vi "Load Project.vi"(8 "error in (no error)":errorcluster, 11 "Application in":refnum<data-value>) -> (0 "error out":errorcluster, 1 "Succeed":bool, 3 "Application out":refnum<data-value>)   [LabVIEW 2015, in "Application.lvclass"]
uses:
  Application.lvclass
  Plugin.lvclass
  Project.lvclass
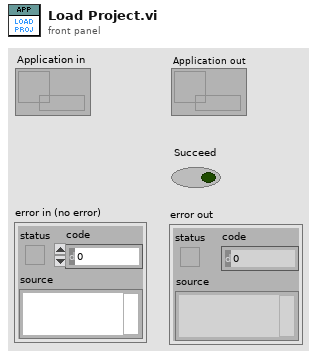
[diagram p1: front panel]
types:
  T1 = typedef "Application Config Typedef.ctl" = cluster{"Auto Load Project":bool, "Project Path":string, "Plugin Folders":string}
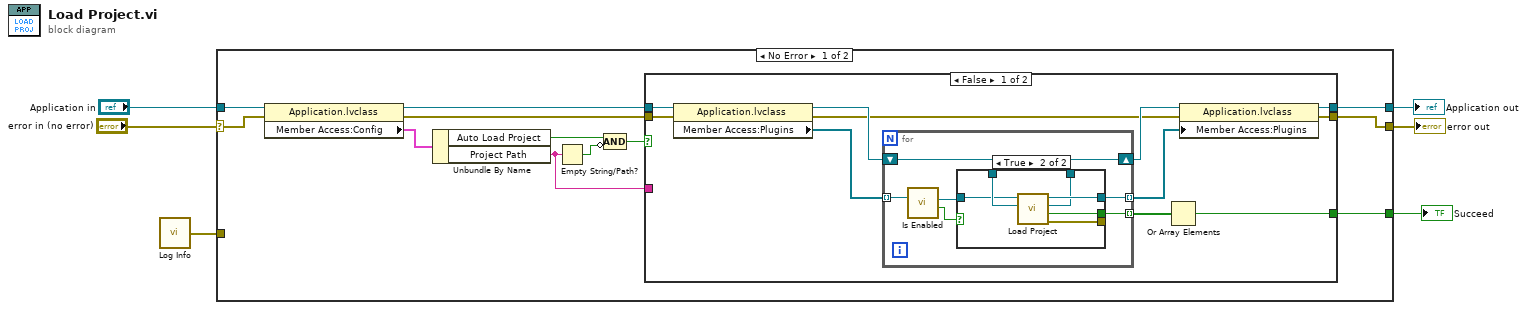
[diagram p0: block diagram]
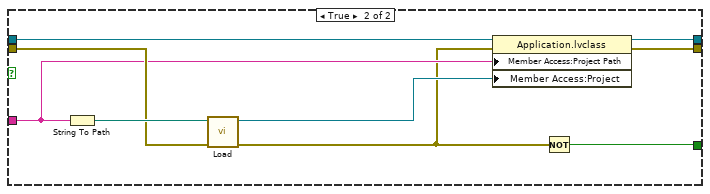
[diagram p3: hidden frame]
diagram:
  n1 = call "Log Info.vi"() -> ("error out"=w4:errorcluster)  [unwired: 5 in]
  n2 = case shown="No Error" "error in (no error)" {
    selector: "error in (no error)" -> [w17 w55]
    tunnel: [w13 w55] -> w5
    tunnel: [w14 w54] -> w2
    tunnel: "Application in" -> [w18 w54]
    tunnel: w4 -> [_ _]
    tunnel: [w12 _] -> w1
    frame No Error {
      n3 = property class="Application.lvclass"(reference=w18, error in=w17) -> (reference out=w16:refnum<data-value>, error out=w15:errorcluster, "Member Access:Config"=w8:T1)
      n4 = Unbundle By Name(w8) -> ("Auto Load Project"=w11:bool, "Project Path"=w7:string)
      n5 = Empty String/Path?(string/path=w7) -> (empty?=w10:bool)
      n6 = Compound Arithmetic op=AND(w11, invert w10) -> (w9:bool)
      n7 = case shown="False" w9 {
        tunnel: w16 -> [w23 w49]
        tunnel: w15 -> [w22 w52]
        tunnel: [w28 w46] -> w14
        tunnel: [w26 w45] -> w13
        tunnel: [w24 w47] -> w12
        tunnel: w7 -> [_ w51]
        frame False {
          n8 = property class="Application.lvclass"(reference=w23, error in=w22) -> (reference out=w20:refnum<data-value>, error out=w19:errorcluster, "Member Access:Plugins"=w21:refnum<class "Plugin.lvclass">[])
          n9 = for {
            tunnel: w21 -> [w32] mode=indexing
            shift-right: [w34] -> w29
            shift-left: w20 -> [w35]
            tunnel: [w36] -> w27 mode=indexing
            tunnel: [w33] -> w25 mode=indexing
            n10 = call "Is Enabled.vi"("Plugin in"=w32) -> ("Enabled"=w30:bool, "Plugin out"=w31:refnum<class "Plugin.lvclass">)  [unwired: 9 in]
            n11 = case shown="True" w30 {
              tunnel: [w38 w44] -> w36
              tunnel: [_ w43] -> _
              tunnel: w35 -> [w37 w42]
              tunnel: [w37 w41] -> w34
              tunnel: [_ w40] -> w33
              tunnel: w31 -> [w38 w39]
              frame False {
              }
              frame True {
                n12 = call-dynamic "Load Project.vi"("Application in"=w42, "Plugin in"=w39) -> ("error out"=w43:errorcluster, "Succeed"=w40:bool, "Application out"=w41:refnum<data-value>, "Plugin out"=w44:refnum<class "Plugin.lvclass">)  [unwired: 6 in]
              }
            }
          }
          n13 = Or Array Elements(Boolean array=w25) -> (logical OR=w24:bool)
          n14 = property class="Application.lvclass"(reference=w29, error in=w19, "Member Access:Plugins"=w27) -> (reference out=w28:refnum<data-value>, error out=w26:errorcluster)
        }
        frame True {
          n15 = String To Path(string=w51) -> (path=w53:path)
          n16 = call "Load.vi"("error in (no error)"=w52, "Project File"=w53) -> ("error out"=w48:errorcluster, "Project"=w50:refnum<class "Project.lvclass">)  [unwired: 8 in]
          n17 = property class="Application.lvclass"(reference=w49, error in=w48, "Member Access:Project Path"=w51, "Member Access:Project"=w50) -> (reference out=w46:refnum<data-value>, error out=w45:errorcluster)
          n18 = Not(x=w48) -> (.not. x?=w47:bool)
        }
      }
    }
    frame Error {
    }
  }
  "error out" <- w5
  "Application out" <- w2
  "Succeed" <- w1
